vi "set_params.vi"(8 "error in (no error)":errorcluster caption="entrée d'erreur (pas d'erreur)", 11 "OrthogonalMatchingPursuit.lvclass 2":refnum<class "OrthogonalMatchingPursuit.lvclass">) -> (0 "error out":errorcluster caption="sortie d'erreur", 3 "OrthogonalMatchingPursuit.lvclass":refnum<class "OrthogonalMatchingPursuit.lvclass">)   [LabVIEW 2020, in "OrthogonalMatchingPursuit.lvclass"]
uses:
  OrthogonalMatchingPursuit.lvclass
  OrthogonalMatchingPursuit.lvclass/OrthogonalMatchingPursuit.ctl
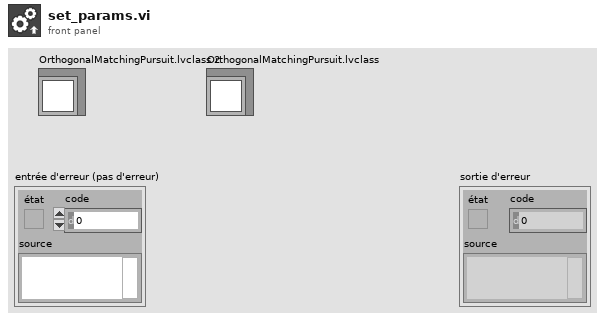
[diagram p1: front panel]
types:
  T1 = typedef "orthogonal_matching_pursuit_params.ctl" = cluster{"n_nonzero_coefs":cluster{"n_nonzero_coefs_type":string, "n_nonzero_coefs_int":dbl}, "tol":cluster{"tol_type":string, "tol_float":dbl}, "fit_intercept":bool, "normalize":bool, "precompute":cluster{"precompute_type":string, "precompute_bool":bool}}
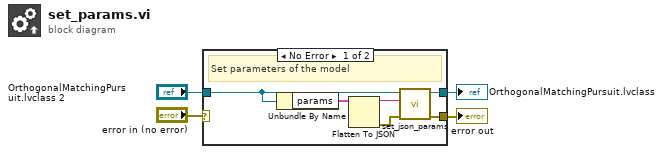
[diagram p0: block diagram]
diagram:
  n1 = case shown="No Error" "error in (no error)" {
    selector: "error in (no error)" -> [_ w12]
    tunnel: [w7 w12] -> w3
    tunnel: [w8 w11] -> w1
    tunnel: "OrthogonalMatchingPursuit.lvclass 2" -> [w5 w11]
    frame No Error {
      # "Set parameters of the model"
      n2 = Unbundle By Name(w5) -> ("params"=w10:T1)
      n3 = Flatten To JSON(anything=w10) -> (JSON string=w9:string, 11:w6:errorcluster)  [unwired: 2 in]
      n4 = call-dynamic "set_json_params.vi"("error in (no error)"=w6, "params"=w9, "Model en entrée"=w5) -> ("error out"=w7:errorcluster, "Model en sortie"=w8:refnum<class "OrthogonalMatchingPursuit.lvclass">)  [unwired: 7 in]
    }
    frame Error {
    }
  }
  "error out" <- w3
  "OrthogonalMatchingPursuit.lvclass" <- w1
